vi "Calculate Home direction.vi"(8 "error in (no error)":errorcluster, 11 "Motor positions":dbl[](array[numeric])) -> (0 "error out":errorcluster, 1 "Home direction M2":T1 items=["", "Forward", "Backward"], 2 "Home direction M1":T1 items=["", "Forward", "Backward"])   [LabVIEW 2025]
uses:
  Public/Controls/Motor direction.ctl
  Control de MaP.lvlib
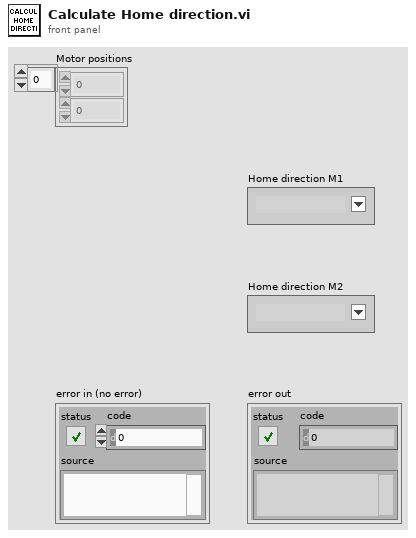
[diagram p1: front panel]
types:
  T1 = typedef "Control de MaP.lvlib/Motor direction.ctl" = u8
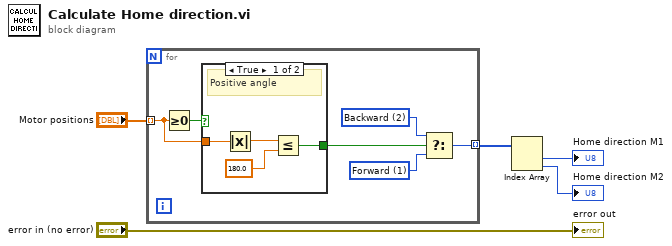
[diagram p0: block diagram]
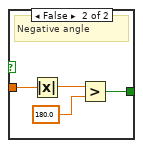
[diagram p2: hidden frame]
diagram:
  n1 = for {
    tunnel: "Motor positions" -> [w10] mode=indexing
    tunnel: [w7] -> w4 mode=indexing
    w8 = T1 1 items=["", "Forward", "Backward"] ("Home direction")
    w9 = T1 2 items=["", "Forward", "Backward"] ("Home direction")
    n2 = Greater Or Equal To 0?(x=w10) -> (x >= 0?=w11:bool)
    n3 = case shown="True" w11 {
      tunnel: w10 -> [w15 w19]
      tunnel: [w12 w16] -> w6
      frame True {
        # "Positive angle"
        n4 = Absolute Value(x=w15) -> (abs(x)=w14:dbl)
        n5 = Less Or Equal?(x=w14, y=180.0) -> (x <= y?=w12:bool)
      }
      frame False {
        # "Negative angle"
        n6 = Absolute Value(x=w19) -> (abs(x)=w18:dbl)
        n7 = Greater?(x=w18, y=180.0) -> (0:w16:bool)
      }
    }
    n8 = Select(t=w9, s=w6, f=w8) -> (s? t:f=w7:T1)
  }
  n9 = Index Array(array=w4) -> (element #1=→"Home direction M1":T1, element #2=→"Home direction M2":T1)  [unwired: 2 in]
  "error out" <- "error in (no error)"
